vi "NichtlinearerRegler2.vi"(10 "x'":dbl=2.0) -> (2 "s? t:f":dbl)   [LabVIEW 2013]
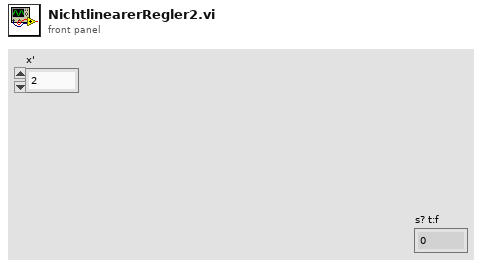
[diagram p1: front panel]
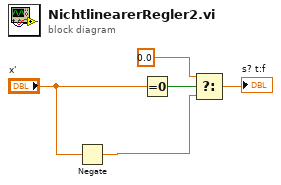
[diagram p0: block diagram]
diagram:
  n1 = Negate(x="x'") -> (-x=w2:dbl)
  n2 = Equal To 0? ("Gleich 0?")(x="x'") -> (x = 0?=w5:bool)
  n3 = Select ("Auswählen")(t=0.0 ("value below threshold 2"), s=w5, f=w2) -> (s? t:f=→"s? t:f":dbl)
